vi "Judge_Arrow.vi"() -> ()   [LabVIEW 2019]
uses:
  WSCbot_V3_Toolkit.lvlibp
panel:
  out "Error Out":errorcluster
  in  "Error In":errorcluster
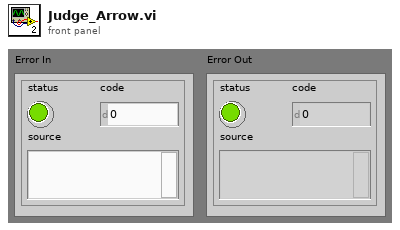
[diagram p1: front panel]
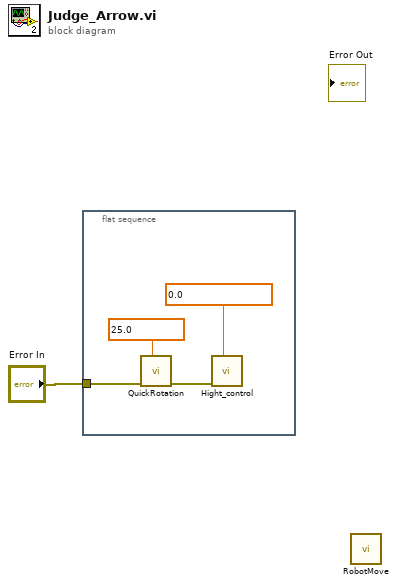
[diagram p0: block diagram]
diagram:
  n1 = flat-sequence {
    tunnel: "Error In" -> [w4]
    frame #0 {
      w2 = 0.0 items=["物料櫃第一格"=0.0, "物料櫃第二格"=78.0, "Á³´U§¨¨ú°ª«×"=128.0, "Á³´UºË·Ç"=250.0, "最高"=288.0] ("Á³±ì°ª«×")
      w5 = 25.0 items=["Forward"=25.0, "Right"=115.0, "Left"=-65.0] ("Á³±ì­±¦V")
      n2 = call "QuickRotation.vi"("Á³±ì­±¦V"=w5, "Error In"=w4) -> ("Error Out"=w3:errorcluster)  [unwired: 9 in]
      n3 = call "Hight_control.vi"("Á³±ì°ª«×"=w2, "Error In"=w3) -> ()  [unwired: 9 in, 1 out]
    }
  }
  n4 = call "RobotMove.vi"() -> ()  [unwired: 11 in, 1 out]
